vi "ping Get Model Num.vi"(8 "error in (no error)":errorcluster, 9 "id":u8, 10 "protocol_version":i32, 11 "port_num":i32) -> (0 "error out":errorcluster, 3 "function return":u16)   [LabVIEW 2018, in "labview.lvlib"]
doc: "WINDECLSPEC uint16_t pingGetModelNum (int port_num, int protocol_version, uint8_t id);"
uses:
  labview.lvlib
  dxl_x86_c.dll
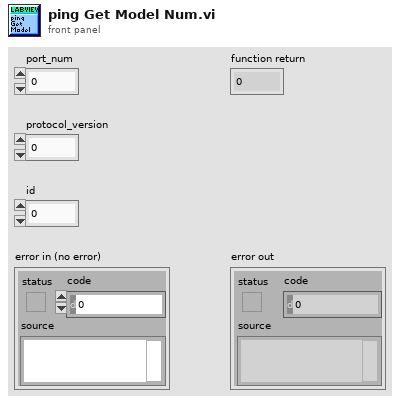
[diagram p1: front panel]
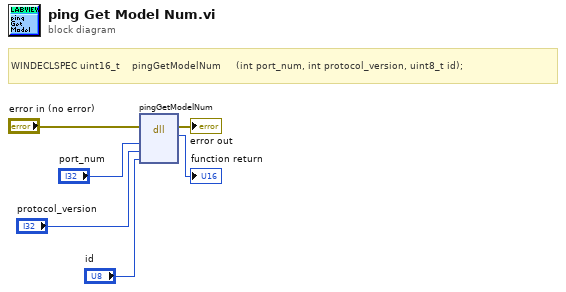
[diagram p0: block diagram]
diagram:
  # "WINDECLSPEC uint16_t    pingGetModelNum     (int port_num, int protocol_version, uint8_t id);"
  n1 = dll-call lib="C:/Users/joaos/OneDrive/Documents/[PhD]/Project Omnidirectional Vehicle/Vanes/LabView_code/joaoandthethreestands/DynamixelSDK-3.7.31/labview/new_compilation/dxl_x86_c.*" fn="pingGetModelNum"(error in="error in (no error)", "port_num"="port_num", "protocol_version"="protocol_version", "id"="id") -> (error out=→"error out":errorcluster, →"function return":u16)  [unwired: 5 in, 1 out]
